vi "SerialCommunication_Demo.vi"(8 "Error In":errorcluster caption="错误输入", 10 "写入":bool, 11 "VISA资源名称":refnum<visa-resource-name>="COM1") -> (0 "Error Out":errorcluster caption="错误输出")   [LabVIEW 2015]
uses:
  <vilib>/Instr/_visa.llb/VISA Configure Serial Port (Instr).vi
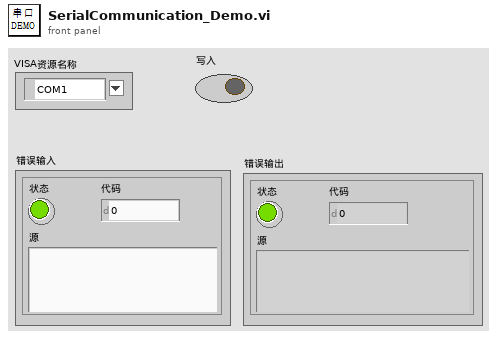
[diagram p1: front panel]
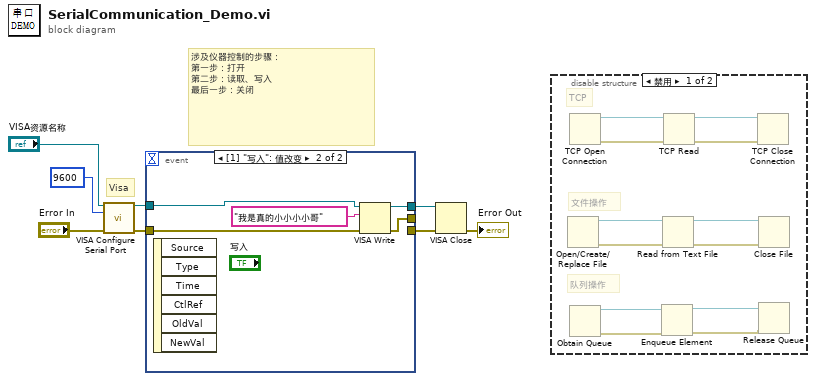
[diagram p0: block diagram]
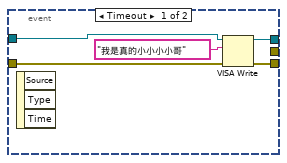
[diagram p2: hidden frame]
diagram:
  # "Visa"
  # "涉及仪器控制的步骤：\n第一步：打开\n第二步：读取、写入\n最后一步：关闭"
  n1 = call-poly "VISA Configure Serial Port"("VISA resource name"="VISA资源名称", "baud rate (9600)"=u32 9600, "error in (no error)"="Error In") -> ("VISA resource name out"=w3:refnum<visa-resource-name>, "error out"=w8:errorcluster)  [unwired: 11 in]
  n2 = event shown="[1] \"写入\": 值改变" {
    selector: _ -> [_ _]
    dyn-events: _ -> [_ _]
    timeout: _ -> [_ _]
    tunnel: w8 -> [w13 w16]
    tunnel: [w12 w15] -> w7
    tunnel: [w11 _] -> w6
    tunnel: w3 -> [w9 w17]
    tunnel: [_ w14] -> _
    event Timeout {
      n3 = event-data() -> ()  [unwired: 1 in, 3 out]
      n4 = VISA Write(VISA resource name=w9, write buffer="我是真的小小小小哥" ("写入缓冲区"), error in (no error)=w13) -> (VISA resource name out=w12:refnum<visa-resource-name>, error out=w11:errorcluster)  [unwired: 1 out]
    }
    event "写入": Value Change {
      n5 = event-data() -> ()  [unwired: 1 in, 6 out]
      n6 = VISA Write(VISA resource name=w17, write buffer="我是真的小小小小哥" ("写入缓冲区"), error in (no error)=w16) -> (VISA resource name out=w15:refnum<visa-resource-name>, error out=w14:errorcluster)  [unwired: 1 out]
    }
  }
  n7 = VISA Close(VISA resource name=w7, error in (no error)=w6) -> (error out=→"Error Out":errorcluster)
  n8 = disable-structure shown="禁用" {
    frame Disabled {
      # "队列操作"
      # "文件操作"
      # "TCP"
      n9 = Open/Create/Replace File() -> (refnum out=w26:refnum<file>, error out=w25:errorcluster)  [unwired: 6 in, 1 out]
      n10 = TCP Open Connection() -> (connection ID=w30:refnum<k5>, error out=w29:errorcluster)  [unwired: 5 in]
      n11 = Obtain Queue() -> (queue out=w22:refnum<queue>, error out=w21:errorcluster)  [unwired: 5 in, 1 out]
      n12 = Enqueue Element(queue=w22, error in (no error)=w21) -> (queue out=w20:refnum<queue>, error out=w19:errorcluster)  [unwired: 2 in, 1 out]
      n13 = Read from Text File(file (use dialog)=w26, error in=w25) -> (refnum out=w24:refnum<file>, error out=w23:errorcluster)  [unwired: 2 in, 2 out]
      n14 = TCP Read(connection ID=w30, error in (no error)=w29) -> (connection ID out=w28:refnum<k5>, error out=w27:errorcluster)  [unwired: 3 in, 1 out]
      n15 = TCP Close Connection(connection ID=w28, error in (no error)=w27) -> ()  [unwired: 1 in, 2 out]
      n16 = Close File(refnum=w24, error in=w23) -> ()  [unwired: 2 out]
      n17 = Release Queue(queue=w20, error in (no error)=w19) -> ()  [unwired: 1 in, 3 out]
    }
    frame Enabled {
    }
  }
